vi "robotWillCollidWithBall.vi"(6 "target":dbl[](array[numeric]) format="%#_13g", 8 "error in (no error)":errorcluster, 9 "Ball":refnum<class "Ball.lvclass">, 10 "Robot":refnum<class "Robot.lvclass">, 11 "Utilities in":refnum<class "Utilities.lvclass">) -> (0 "error out":errorcluster, 2 "robotCollideWithBall":bool, 3 "Utilities out":refnum<class "Utilities.lvclass">)   [LabVIEW 2023, in "Utilities.lvclass"]
uses:
  Utilities.lvclass
  Robot_class/Robot.lvclass
  C:/Users/ebert/Desktop/roboime/SSL_AI/Object_class/Object.lvclass
  Ball_class/Ball.lvclass
  Object_class/Object.lvclass/Object.ctl
  <vilib>/Analysis/coordinate.llb/2D Cartesian Coordinate Rotation (Scalar).vi
  Object_class/Read position(x,y).vi
  Object_class/Read y.vi
  Object_class/Read x.vi
  <vilib>/Analysis/NI_AALPro.lvlib
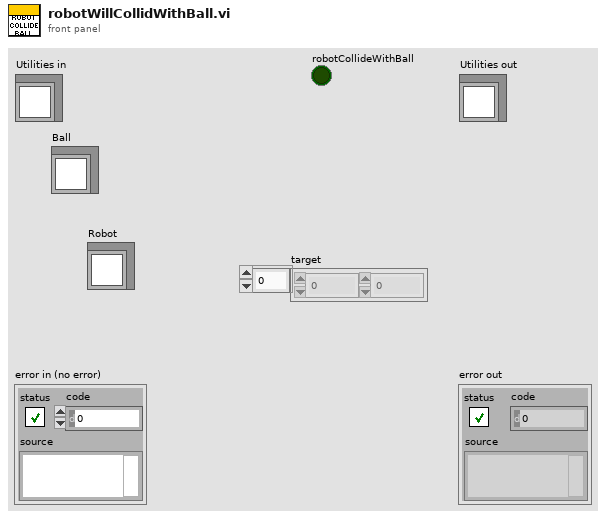
[diagram p1: front panel]
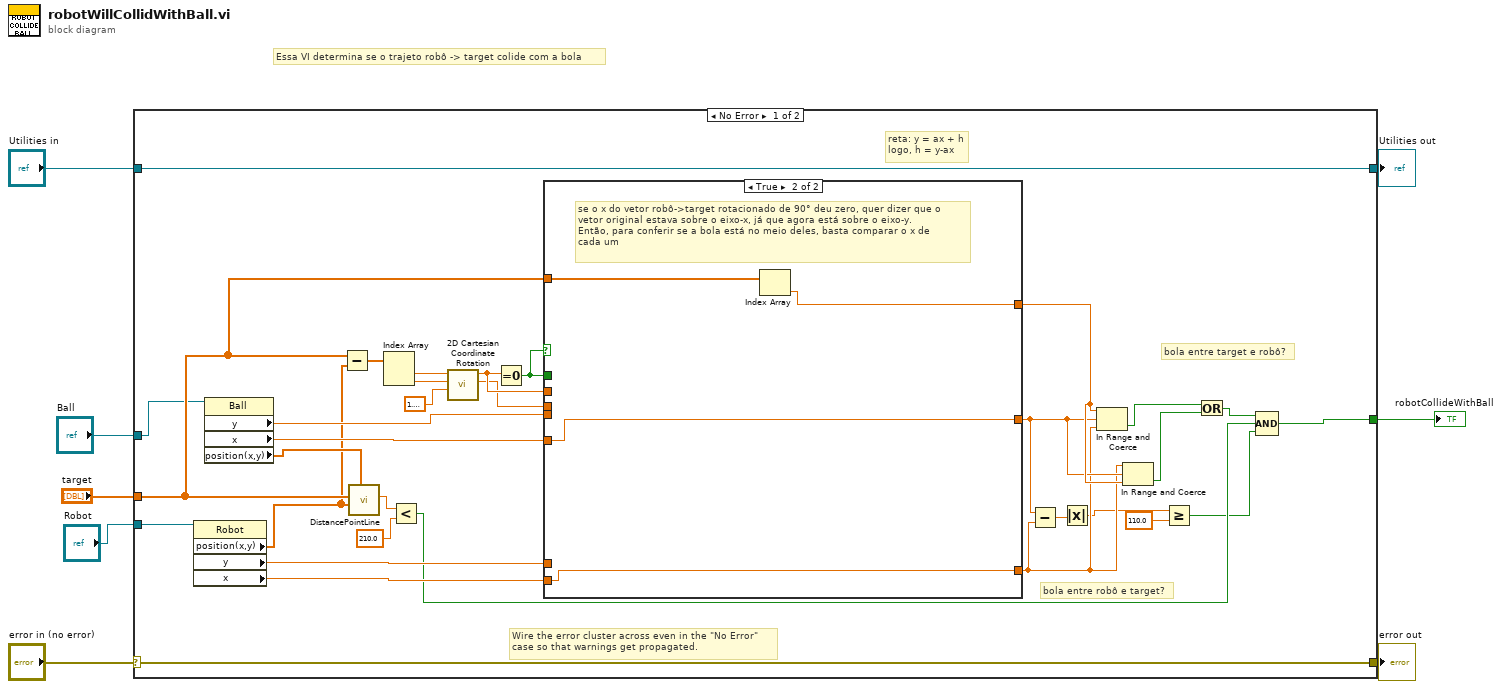
[diagram p0: block diagram]
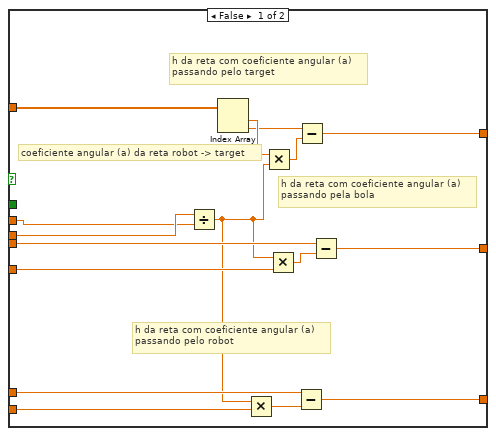
[diagram p2: hidden frame]
diagram:
  # "Essa VI determina se o trajeto robô -> target colide com a bola"
  n1 = case shown="No Error" "error in (no error)" {
    selector: "error in (no error)" -> [w39 w62]
    tunnel: [w39 w62] -> w7
    tunnel: [w40 w61] -> w5
    tunnel: "Utilities in" -> [w40 w61]
    tunnel: "Ball" -> [w17 _]
    tunnel: "target" -> [w30 _]
    tunnel: "Robot" -> [w16 _]
    tunnel: [w20 _] -> w1
    frame No Error {
      # "bola entre target e robô?"
      # "bola entre robô e target?"
      # "reta: y = ax + h\nlogo, h = y-ax"
      # "Wire the error cluster across even in the \"No Error\"\ncase so that warnings get propagated."
      n2 = property class="Robot"(reference=w16) -> ("position(x,y)"=w18:dbl[], "y"=w27:dbl, "x"=w26:dbl)  [unwired: 1 in, 2 out]
      n3 = property class="Ball"(reference=w17) -> ("y"=w29:dbl, "x"=w28:dbl, "position(x,y)"=w19:dbl[])  [unwired: 1 in, 2 out]
      n4 = Subtract(x=w30, y=w18) -> (x-y=w36:dbl[])
      n5 = call "DistancePointLine.vi"("Q"=w19, "P2"=w18, "P1"=w30) -> ("distance"=w38:dbl)  [unwired: 5 in, 3 out]
      n6 = Index Array(array=w36) -> (element #1=w35:dbl, element #2=w34:dbl)  [unwired: 2 in]
      n7 = Less?(x=w38, y=210.0) -> (x < y?=w21:bool)
      n8 = call-poly <vilib>:"2D Cartesian Coordinate Rotation.vi"("theta"=1.5707963267948966, "y"=w34, "x"=w35) -> ("y out"=w31:dbl, "x out"=w32:dbl)  [unwired: 6 in, 1 out]
      n9 = Equal To 0?(x=w32) -> (x = 0?=w15:bool)
      n10 = case shown="True" w15 {
        tunnel: w15 -> [_ _]
        tunnel: w32 -> [w41 _]
        tunnel: w31 -> [w56 _]
        tunnel: w30 -> [w55 w60]
        tunnel: w29 -> [w50 _]
        tunnel: w28 -> [w49 w58]
        tunnel: w27 -> [w48 _]
        tunnel: w26 -> [w47 w57]
        tunnel: [w44 w58] -> w14
        tunnel: [w43 w57] -> w13
        tunnel: [w42 w59] -> w24
        frame False {
          # "h da reta com coeficiente angular (a)\npassando pela bola"
          # "h da reta com coeficiente angular (a)\npassando pelo robot"
          # "h da reta com coeficiente angular (a)\npassando pelo target"
          # "coeficiente angular (a) da reta robot -> target"
          n11 = Divide(x=w56, y=w41) -> (x/y=w46:dbl)
          n12 = Index Array(array=w55) -> (element #1=w54:dbl, element #2=w53:dbl)  [unwired: 2 in]
          n13 = Multiply(x=w46, y=w47) -> (x*y=w45:dbl)
          n14 = Multiply(x=w54, y=w46) -> (x*y=w52:dbl)
          n15 = Multiply(x=w46, y=w49) -> (x*y=w51:dbl)
          n16 = Subtract(x=w48, y=w45) -> (x-y=w43:dbl)
          n17 = Subtract(x=w53, y=w52) -> (x-y=w42:dbl)
          n18 = Subtract(x=w50, y=w51) -> (x-y=w44:dbl)
        }
        frame True {
          # "se o x do vetor robô->target rotacionado de 90° deu zero, quer dizer que o\nvetor original estava sobre o eixo-x, já que agora está sobre o eixo-y.\nEntão, para conferir se a bola está no meio deles, basta comparar o x de\ncada um"
          n19 = Index Array(array=w60) -> (element=w59:dbl)  [unwired: 1 in]
        }
      }
      n20 = Subtract(x=w14, y=w13) -> (x-y=w12:dbl)
      n21 = Absolute Value(x=w12) -> (abs(x)=w11:dbl)
      n22 = In Range and Coerce(upper limit=w24, x=w14, lower limit=w13) -> (In Range?=w25:bool)  [unwired: 1 out]
      n23 = In Range and Coerce(upper limit=w13, x=w14, lower limit=w24) -> (In Range?=w23:bool)  [unwired: 1 out]
      n24 = Greater Or Equal?(x=w11, y=110.0) -> (x >= y?=w9:bool)
      n25 = Or(x=w25, y=w23) -> (x .or. y?=w22:bool)
      n26 = Compound Arithmetic op=AND(w22, w21, w9) -> (w20:bool)
    }
    frame Error {
    }
  }
  "error out" <- w7
  "Utilities out" <- w5
  "robotCollideWithBall" <- w1
